vi "MotionCharacterization.vi"() -> ()   [LabVIEW 2014]
panel:
  out "Error":dbl(graph)
  out "Pose":cluster{"X":dbl, "Y":dbl}[](array[cluster])
  out "Detected Location":cluster{"X":dbl, "Y":dbl}[](graph)
  out "Avg. Search Time":dbl(knob) scale=0.0..5000.0
  out "Data Valid?":bool
  out "Search Timing":u32(graph)
  in  "stop":bool
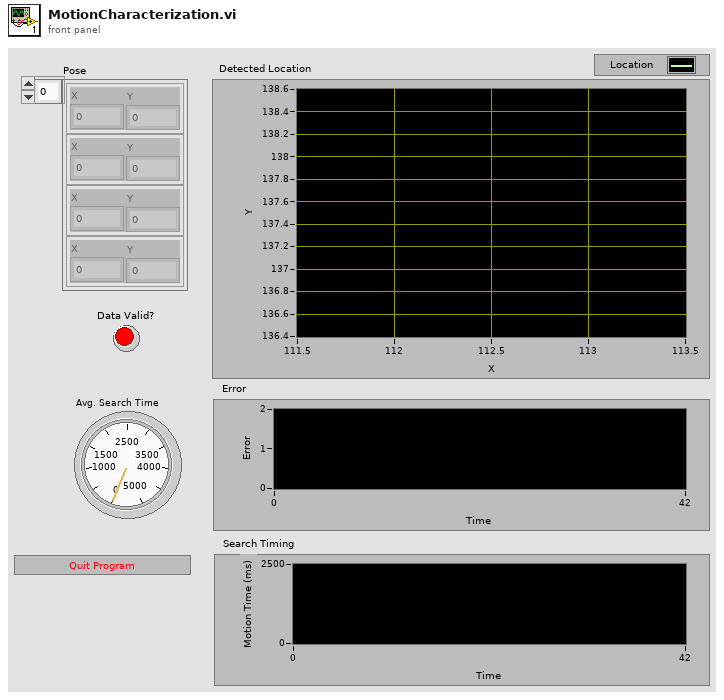
[diagram p1: front panel]
types:
  T1 = enum16{"Standard", "Buffered", "CRLF", "Immediate"}
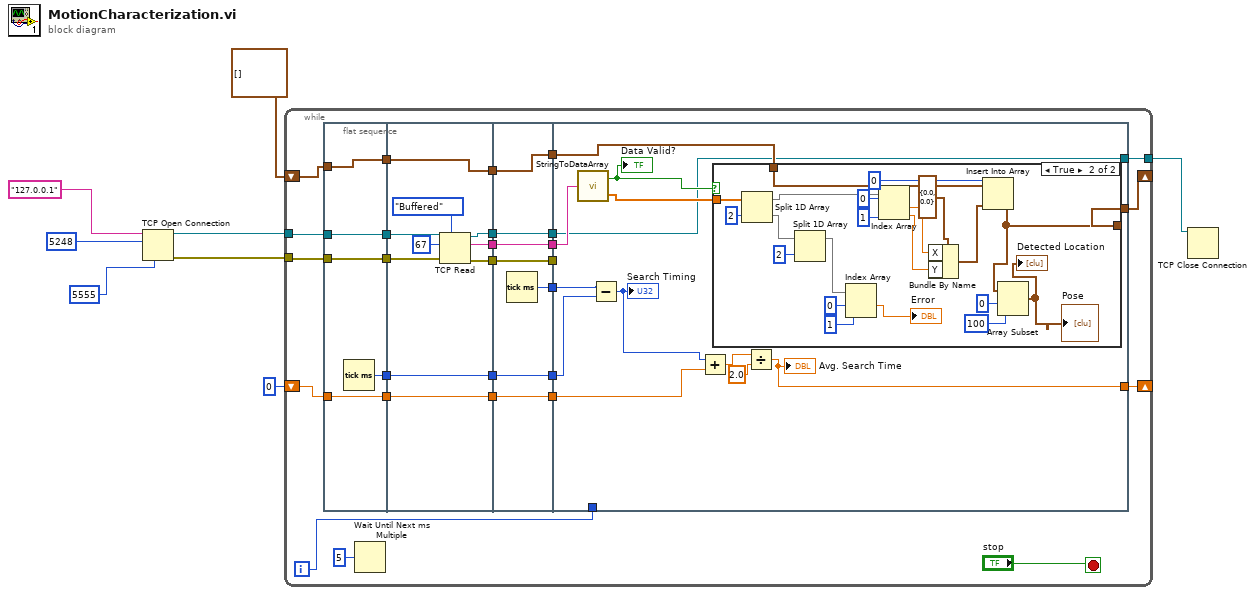
[diagram p0: block diagram]
diagram:
  n1 = TCP Open Connection(address="127.0.0.1", remote port or service name=u16 5248, local port=u16 5555 ("local port (0)")) -> (connection ID=w8:refnum<k5>, error out=w7:errorcluster)  [unwired: 2 in]
  n2 = while {
    tunnel: w8 -> [w18]
    tunnel: w7 -> [w17]
    shift-right: [w23] -> _
    shift-left: u32 0 -> [w19]
    tunnel: [w12] -> w1
    shift-right: [w9] -> _
    shift-left: cluster{"X":dbl, "Y":dbl}[] [] ("XY Graph") -> [w13]
    i -> [w24]
    stop <- "stop" stop-if-true
    n3 = flat-sequence {
      tunnel: [w39] -> w34
      tunnel: [w38] -> w33
      tunnel: [w41] -> w26
      tunnel: [w40] -> w20
      tunnel: w19 -> [w40]
      tunnel: w18 -> [w39]
      tunnel: w17 -> [w38]
      tunnel: [w37] -> w14
      tunnel: w13 -> [w37]
      tunnel: w34 -> [w51]
      tunnel: w33 -> [w50]
      tunnel: [w49] -> w31
      tunnel: [w48] -> w29
      tunnel: [w47] -> w27
      tunnel: w26 -> [w47]
      tunnel: [w44] -> w21
      tunnel: w20 -> [w44]
      tunnel: [w43] -> w15
      tunnel: w14 -> [w43]
      tunnel: [w42] -> w10
      tunnel: [w58] -> w32
      tunnel: w31 -> [w58]
      tunnel: [w55] -> w30
      tunnel: w29 -> [w55]
      tunnel: [w57] -> w28
      tunnel: w27 -> [w57]
      tunnel: [w56] -> w25
      tunnel: [w54] -> w22
      tunnel: w21 -> [w54]
      tunnel: [w53] -> w16
      tunnel: w15 -> [w53]
      tunnel: [w52] -> w11
      tunnel: w10 -> [w52]
      tunnel: w32 -> [_]
      tunnel: w30 -> [w69]
      tunnel: w28 -> [w70]
      tunnel: w25 -> [w71]
      tunnel: w24 -> [_]
      tunnel: [w62] -> w23
      tunnel: w22 -> [w66]
      tunnel: w16 -> [w61]
      tunnel: [w60] -> w12
      tunnel: w11 -> [w60]
      tunnel: [w59] -> w9
      frame #0 {
        n4 = Tick Count (ms)() -> (millisecond timer value=w41:u32)
      }
      frame #1 {
        n5 = TCP Read(connection ID=w51, bytes to read=67, error in (no error)=w50, 7:T1."Buffered" ("mode (standard)")) -> (connection ID out=w42:refnum<k5>, data out=w48:string, error out=w49:errorcluster)  [unwired: 1 in]
      }
      frame #2 {
        n6 = Tick Count (ms)() -> (millisecond timer value=w56:u32)
      }
      frame #3 {
        n7 = call "StringToDataArray.vi"("Data In"=w69) -> ("Good Data"=w67:bool, "Data Out"=w68:dbl[])
        "Data Valid?" <- w67
        n8 = Subtract(x=w71, y=w70) -> (x-y=w65:u32)
        "Search Timing" <- w65
        n9 = Add(x=w65, y=w66) -> (x+y=w63:dbl)
        n10 = case shown="True" w67 {
          tunnel: w68 -> [_ w93]
          tunnel: w61 -> [w72 w89]
          tunnel: [w72 w80] -> w59
          frame False {
          }
          frame True {
            n11 = Split 1D Array(array=w93, index=2) -> (first subarray=w88:dbl[], second subarray=w91:dbl[])
            n12 = Split 1D Array(array=w91, index=2) -> (first subarray=w76:dbl[])  [unwired: 1 out]
            n13 = Index Array(array=w76, index #1=0 ("index"), index #2=1 ("index")) -> (element #1=→"Error":dbl)  [unwired: 1 out]
            n14 = Index Array(array=w88, index #1=0 ("index"), index #2=1 ("index")) -> (element #1=w85:dbl, element #2=w84:dbl)
            n15 = Bundle By Name(cluster=cluster{"X":dbl, "Y":dbl} {"X"=0.0, "Y"=0.0} ("new element/subarray"), "X"=w85, "Y"=w84) -> (w82:cluster{"X":dbl, "Y":dbl})
            n16 = Insert Into Array(array=w89, index=0, new element=w82) -> (w80:cluster{"X":dbl, "Y":dbl}[])
            n17 = Array Subset(array=w80, index=0, length=100) -> (→"Detected Location" →"Pose":cluster{"X":dbl, "Y":dbl}[])
          }
        }
        n18 = Divide(x=w63, y=2.0) -> (x/y=w62:dbl)
        "Avg. Search Time" <- w62
      }
    }
    n19 = Wait Until Next ms Multiple(millisecond multiple=u32 5) -> ()  [unwired: 1 out]
  }
  n20 = TCP Close Connection(connection ID=w1) -> ()  [unwired: 2 in, 2 out]
